vi "tm430_functions_41.vi"() -> ()   [LabVIEW 2023, in "HamamatsuCam.lvlib" / "HamamatsuCam.lvclass"]
uses:
  HamamatsuCam/HamamatsuCam/HamamatsuCam.lvclass
panel:
  in  "View":dbl min=1.0 max=1.0 step=1.0
  out "Image":u16[][](graph)
  in  "Snap":bool
  in  "Parameter":u32(ring)=4212128 items=["SENSOR MODE"=4212128, "SENSOR MODE LINE BUNDLE HEIGHT"=4212192, "BIT PER CHANNEL"=4342976, "TRIGGER ENABLE ACTIVE"=1066912, "TRIGGER ENABLE POLARITY"=1066928, "TRIGGER NUMBER FOR FIRST IMAGE"=1067936, "TRIGGER NUMBER FOR NEXT IMAGE"=1067952, "EXPOSURE TIME"=2049184, "TAPCALIB GAIN[0]"=3691408, "TAPCALIB GAIN[1]"=3691424, "TAPCALIB GAIN[2]"=3691440, "TAPCALIB GAIN[3]"=3691456, "TAPCALIB GAIN[4]"=3691472, "TAPCALIB GAIN[5]"=3691488, "TAPCALIB GAIN[6]"=3691504, "TAPCALIB GAIN[7]"=3691520, "TAPCALIB GAIN[8]"=3691536, "TAPCALIB GAIN[9]"=3691552, "TAPCALIB GAIN[10]"=3691568, "TAPCALIB GAIN[11]"=3691584, "DEFECT CORRECT MODE"=4670368, "BINNING"=4215968, "BINNING INDEPENDENT"=4215984, "BINNING HORZ"=4216000, "BINNING VERT"=4216016, "INTERNAL FRAME RATE"=4225952, "INTERNAL FRAME INTERVAL"=4225968, "INTERNAL LINE SPEED"=4226000, "IMAGE WIDTH"=4343200, "IMAGE HEIGHT"=4343216, "IMAGE ROWBYTES"=4343232, "IMAGE FRAMEBYTES"=4343248, "IMAGE PIXEL TYPE"=4343296]
  in  "Text Value":dbl(ring)
  in  "Value":dbl(slide) min=0.0 max=63.0 step=1.0 scale=1.0..2.0
  out "error out":errorcluster
  in  "stop":bool
  # "This example shows a way you can access\nmany of the functions available to the camera and see how they affect the captured image."
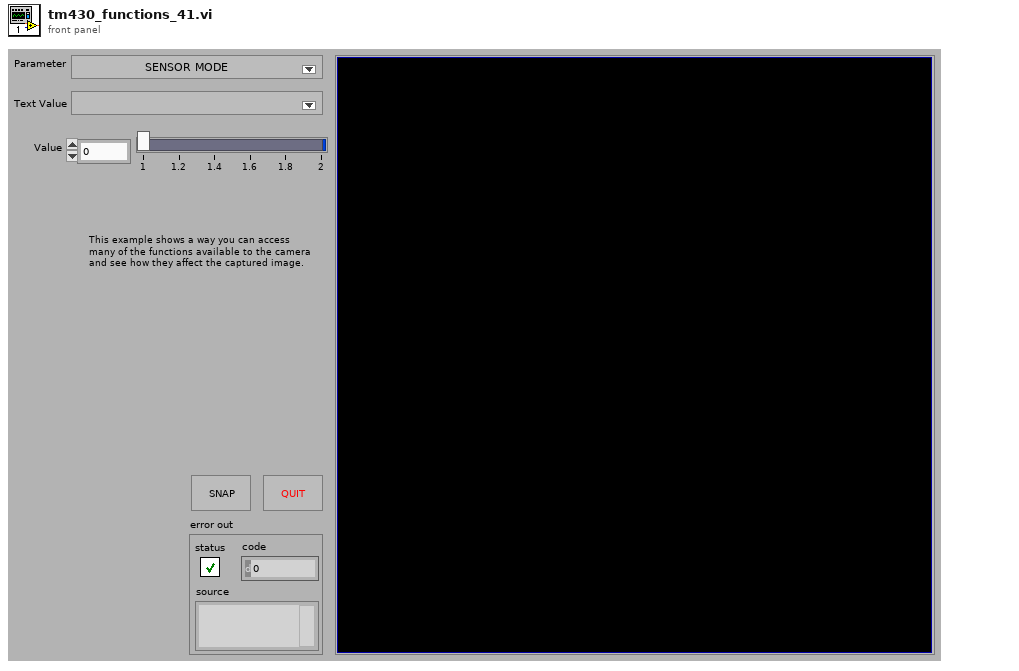
[diagram p1: front panel]
types:
  T1 = enum8{"Enabled", "Disabled", "Disabled and Grayed Out"}
  T2 = cluster{"Function Name":string, "Function ID":u32}[]
  T3 = cluster{"Function Name":string, "Function ID":u32}
  T4 = cluster{"Range":cluster{"min":dbl, "max":dbl, "step":dbl}, "default":dbl, "views":u32, "Writable":bool, "Text Values":bool, "Value Names":cluster{"Name":string, "Value":dbl}[]}
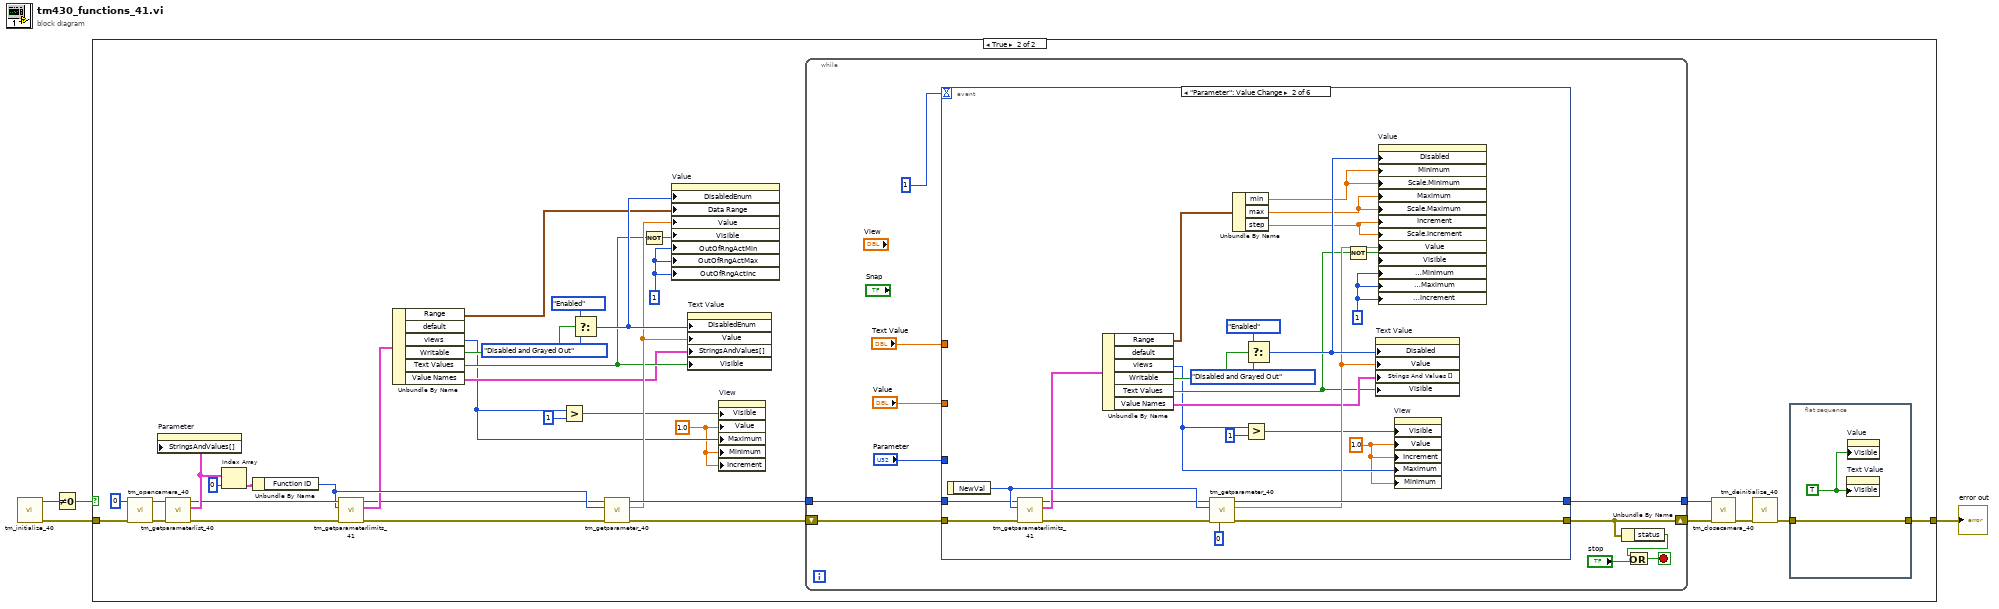
[diagram p0: block diagram]
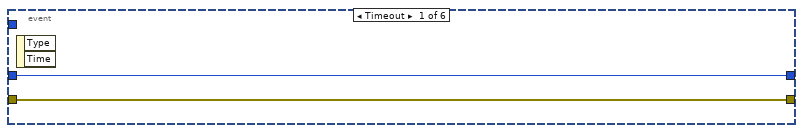
[diagram p3: hidden frame]
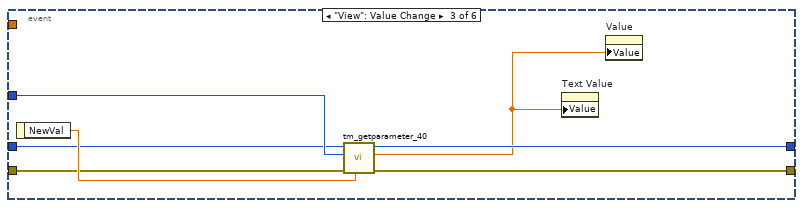
[diagram p4: hidden frame]
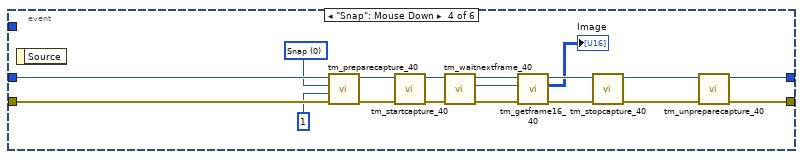
[diagram p5: hidden frame]
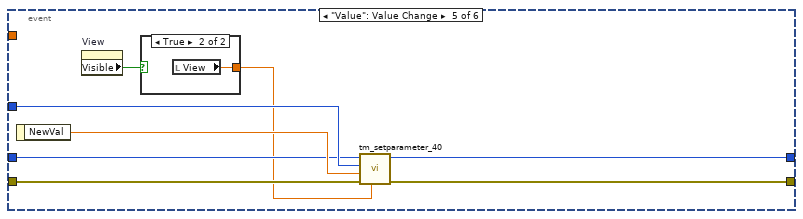
[diagram p6: hidden frame]
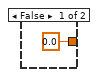
[diagram p7: hidden frame]
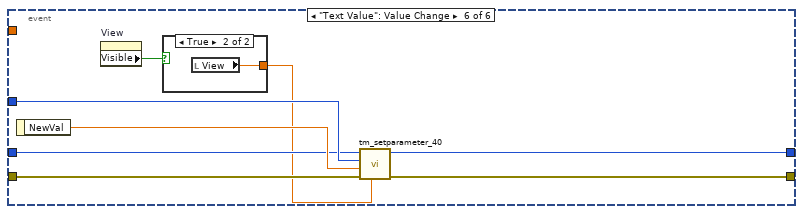
[diagram p8: hidden frame]
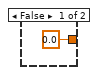
[diagram p9: hidden frame]
diagram:
  n1 = call "tm_initialize_40.vi"() -> ("error out"=w2:errorcluster, "Number Of Cameras"=w4:u32)  [unwired: 8 in, 2 out]
  n2 = Not Equal To 0?(x=w4) -> (x != 0?=w3:bool)
  n3 = case shown="True" w3 {
    tunnel: [w5 w34] -> w1
    tunnel: w2 -> [w5 w39]
    frame False {
    }
    frame True {
      w6 = 1.0 ("View")
      w26 = u8 1 ("Out Of Range Action:Increment")
      n4 = call "tm_opencamera_40.vi"("error in (no error)"=w39, "Camera Index"=u32 0) -> ("error out"=w36:errorcluster, "Handle out"=w37:u32)  [unwired: 7 in, 1 out]
      n5 = call "tm_getparameterlist_40.vi"("error in (no error)"=w36, "Handle in"=w37) -> ("error out"=w17:errorcluster, "Function List"=w22:T2, "Handle out"=w19:u32)  [unwired: 7 in]
      n6 = property on="Parameter" class="Ring (strict)"("StringsAndValues[]"=w22) -> ()  [unwired: 2 in, 2 out]
      n7 = Index Array(array=w22, index=0) -> (element=w20:T3)
      n8 = Unbundle By Name(w20) -> ("Function ID"=w18:u32)
      n9 = call "tm_getparameterlimits_41.vi"("error in (no error)"=w17, "Parameter"=w18, "Handle in"=w19) -> ("error out"=w11:errorcluster, "Limits"=w16:T4, "Handle out"=w10:u32)  [unwired: 6 in]
      n10 = Unbundle By Name(w16) -> ("Range"=w15:cluster{"min":dbl, "max":dbl, "step":dbl}, "views"=w7:u32, "Writable"=w14:bool, "Text Values"=w13:bool, "Value Names"=w12:cluster{"Name":string, "Value":dbl}[])  [unwired: 1 out]
      n11 = Greater?(x=w7, y=u32 1) -> (0:w8:bool)
      n12 = Select(t=T1."Enabled" ("Disabled"), s=w14, f=T1."Disabled and Grayed Out" ("Disabled")) -> (s? t:f=w28:T1)
      n13 = call "tm_getparameter_40.vi"("error in (no error)"=w11, "Parameter"=w18, "Handle in"=w10) -> ("error out"=w23:errorcluster, "Value out"=w24:dbl, "Handle out"=w25:u32)  [unwired: 6 in]
      n14 = Not(x=w13) -> (.not. x?=w27:bool)
      n15 = property on="Value" class="Slide (strict)"("DisabledEnum"=w28, "Data Range"=w15, "Value"=w24, "Visible"=w27, "OutOfRngActMin"=w26, "OutOfRngActMax"=w26, "OutOfRngActInc"=w26) -> ()  [unwired: 2 in, 2 out]
      n16 = property on="Text Value" class="Ring (strict)"("DisabledEnum"=w28, "Value"=w24, "StringsAndValues[]"=w12, "Visible"=w13) -> ()  [unwired: 2 in, 2 out]
      n17 = property on="View" class="DigNum (strict)"("Visible"=w8, "Value"=w6, "Maximum"=w7, "Minimum"=w6, "Increment"=w6) -> ()  [unwired: 2 in, 2 out]
      n18 = while {
        tunnel: w25 -> [w48]
        tunnel: [w46] -> w32
        shift-right: [w45] -> w33
        shift-left: w23 -> [w49]
        stop <- w50 stop-if-true
        n19 = event shown="[1] \"Parameter\": Value Change" {
          selector: _ -> [_ _ _ _ _ _]
          dyn-events: _ -> [_ _ _ _ _ _]
          timeout: 1 -> [_ _ _ _ _ _]
          tunnel: w49 -> [w54 w70 w81 w104 w113 w123]
          tunnel: w48 -> [w53 w71 w82 w105 w110 w119]
          tunnel: [w53 w75 w87 w95 w109 w118] -> w46
          tunnel: [w54 w73 w85 w94 w108 w122] -> w45
          tunnel: "Parameter" -> [_ _ w84 _ w111 w120]
          tunnel: "Value" -> [_ _ _ _ _ _]
          tunnel: "Text Value" -> [_ _ _ _ _ _]
          event Timeout {
            n20 = event-data() -> ()  [unwired: 1 in, 2 out]
          }
          event "Parameter": Value Change {
            w59 = 1.0 ("View")
            w79 = u8 1 ("Out Of Range Action:Increment")
            n21 = event-data() -> ("NewVal"=w72:u32)  [unwired: 1 in]
            n22 = call "tm_getparameterlimits_41.vi"("error in (no error)"=w70, "Parameter"=w72, "Handle in"=w71) -> ("error out"=w67:errorcluster, "Limits"=w69:T4, "Handle out"=w68:u32)  [unwired: 6 in]
            n23 = Unbundle By Name(w69) -> ("Range"=w58:cluster{"min":dbl, "max":dbl, "step":dbl}, "views"=w60:u32, "Writable"=w66:bool, "Text Values"=w64:bool, "Value Names"=w65:cluster{"Name":string, "Value":dbl}[])  [unwired: 1 out]
            n24 = call "tm_getparameter_40.vi"("Index"=0, "error in (no error)"=w67, "Parameter"=w72, "Handle in"=w68) -> ("error out"=w73:errorcluster, "Value out"=w74:dbl, "Handle out"=w75:u32)  [unwired: 5 in]
            n25 = Unbundle By Name(w58) -> ("min"=w57:dbl, "max"=w56:dbl, "step"=w55:dbl)
            n26 = Greater?(x=w60, y=u32 1) -> (0:w62:bool)
            n27 = Select(t=T1."Enabled" ("Disabled"), s=w66, f=T1."Disabled and Grayed Out" ("Disabled")) -> (s? t:f=w78:T1)
            n28 = Not(x=w64) -> (.not. x?=w80:bool)
            n29 = property on="Text Value" class="Ring (strict)"("Disabled"=w78, "Value"=w74, "Strings And Values []"=w65, "Visible"=w64) -> ()  [unwired: 2 in, 2 out]
            n30 = property on="Value" class="Slide (strict)"("Disabled"=w78, "Minimum"=w57, "Scale.Minimum"=w57, "Maximum"=w56, "Scale.Maximum"=w56, "Increment"=w55, "Scale.Increment"=w55, "Value"=w74, "Visible"=w80, "Response to Value Outside Limits:Minimum"=w79, "Response to Value Outside Limits:Maximum"=w79, "Response to Value Outside Limits:Increment"=w79) -> ()  [unwired: 2 in, 2 out]
            n31 = property on="View" class="DigNum (strict)"("Visible"=w62, "Value"=w59, "Increment"=w59, "Maximum"=w60, "Minimum"=w59) -> ()  [unwired: 2 in, 2 out]
          }
          event "View": Value Change {
            n32 = event-data() -> ("NewVal"=w83:dbl)  [unwired: 1 in]
            n33 = call "tm_getparameter_40.vi"("Index"=w83, "error in (no error)"=w81, "Parameter"=w84, "Handle in"=w82) -> ("error out"=w85:errorcluster, "Value out"=w86:dbl, "Handle out"=w87:u32)  [unwired: 5 in]
            n34 = property on="Text Value" class="Ring (strict)"("Value"=w86) -> ()  [unwired: 2 in, 2 out]
            n35 = property on="Value" class="Slide (strict)"("Value"=w86) -> ()  [unwired: 2 in, 2 out]
          }
          event "Snap": Mouse Down {
            w103 = 0 items=["Snap", "Sequence"] ("Capture mode")
            n36 = event-data() -> ()  [unwired: 1 in, 1 out]
            n37 = call "tm_preparecapture_40.vi"("error in (no error)"=w104, "Frames"=1, "Capture mode"=w103, "Handle in"=w105) -> ("error out"=w101:errorcluster, "Handle out"=w100:u32)  [unwired: 4 in, 2 out]
            n38 = call "tm_startcapture_40.vi"("error in (no error)"=w101, "Handle in"=w100) -> ("error out"=w92:errorcluster, "Handle out"=w93:u32)  [unwired: 8 in]
            n39 = call "tm_waitnextframe_40.vi"("error in (no error)"=w92, "Handle in"=w93) -> ("error out"=w90:errorcluster, "Frame Index"=w88:i32, "Handle out"=w91:u32)  [unwired: 6 in, 1 out]
            n40 = call "tm_getframe16_40.vi"("error in (no error)"=w90, "Frame Index"=w88, "Handle in"=w91) -> ("error out"=w98:errorcluster, "Data"=→"Image":u16[][], "Handle out"=w99:u32)  [unwired: 5 in, 1 out]
            n41 = call "tm_stopcapture_40.vi"("error in (no error)"=w98, "Handle in"=w99) -> ("error out"=w97:errorcluster, "Handle out"=w96:u32)  [unwired: 8 in]
            n42 = call "tm_unpreparecapture_40.vi"("error in (no error)"=w97, "Handle in"=w96) -> ("error out"=w94:errorcluster, "Handle out"=w95:u32)  [unwired: 8 in]
          }
          event "Value": Value Change {
            n43 = event-data() -> ("NewVal"=w112:dbl)  [unwired: 1 in]
            n44 = property on="View" class="DigNum (strict)"() -> ("Visible"=w107:bool)  [unwired: 2 in, 2 out]
            n45 = case shown="True" w107 {
              tunnel: [0.0 ("View") w115] -> w106
              frame False {
              }
              frame True {
                n46 = local read "View"() -> (w115:dbl)
              }
            }
            n47 = call "tm_setparameter_40.vi"("Index"=w106, "error in (no error)"=w113, "Value in"=w112, "Parameter"=w111, "Handle in"=w110) -> ("error out"=w108:errorcluster, "Handle out"=w109:u32)  [unwired: 5 in]
          }
          event "Text Value": Value Change {
            n48 = event-data() -> ("NewVal"=w121:dbl)  [unwired: 1 in]
            n49 = property on="View" class="DigNum (strict)"() -> ("Visible"=w117:bool)  [unwired: 2 in, 2 out]
            n50 = case shown="True" w117 {
              tunnel: [0.0 ("View") w125] -> w116
              frame False {
              }
              frame True {
                n51 = local read "View"() -> (w125:dbl)
              }
            }
            n52 = call "tm_setparameter_40.vi"("Index"=w116, "error in (no error)"=w123, "Value in"=w121, "Parameter"=w120, "Handle in"=w119) -> ("error out"=w122:errorcluster, "Handle out"=w118:u32)  [unwired: 5 in]
          }
        }
        n53 = Unbundle By Name(w45) -> ("status"=w51:bool)
        n54 = Or(x=w51, y="stop") -> (x .or. y?=w50:bool)
      }
      n55 = call "tm_closecamera_40.vi"("error in (no error)"=w33, "Handle in"=w32) -> ("error out"=w38:errorcluster)  [unwired: 9 in]
      n56 = call "tm_deinitialize_40.vi"("error in (no error)"=w38) -> ("error out"=w35:errorcluster)  [unwired: 10 in]
      n57 = flat-sequence {
        tunnel: w35 -> [w41]
        tunnel: [w41] -> w34
        frame #0 {
          w40 = TRUE
          n58 = property on="Text Value" class="Ring (strict)"("Visible"=w40) -> ()  [unwired: 2 in, 2 out]
          n59 = property on="Value" class="Slide (strict)"("Visible"=w40) -> ()  [unwired: 2 in, 2 out]
        }
      }
    }
  }
  "error out" <- w1
